vi "POP_Point to Row Col.vi"(8 "error in (no error)":errorcluster, 9 "Point":cluster{"X":i32, "Y":i32}, 11 "Grid Ctl Reference In":refnum<vi>) -> (0 "error out":errorcluster, 1 "Cell Rect Out":T3={"left"=28, "top"=253, "right"=88, "bottom"=213}, 2 "Cell Info Out":T1={"Tag"="", "Row"=0, "Column"=0, "In Symbol?"=FALSE, "In Data?"=FALSE, "Cell String"="", "Ctl Refnum"=refnum, "Prop Type"=enum."Unkown", "Ring Strings"=[], "Ring Values"=[], "New Cell String"=""}, 3 "Grid Ctl Reference Out":refnum<vi>, 4 "In Bounds?":bool)   [LabVIEW 2016]
uses:
  Ctrls/PSPOP_Grid.Cell Info.ctl
  Ctrls/POP_Data Type.ctl
panel:
  in  "Cell Info (type)":T1={"Tag"="", "Row"=0, "Column"=0, "In Symbol?"=FALSE, "In Data?"=FALSE, "Cell String"="", "Ctl Refnum"=refnum, "Prop Type"=enum."Unkown", "Ring Strings"=[], "Ring Values"=[], "New Cell String"=""}
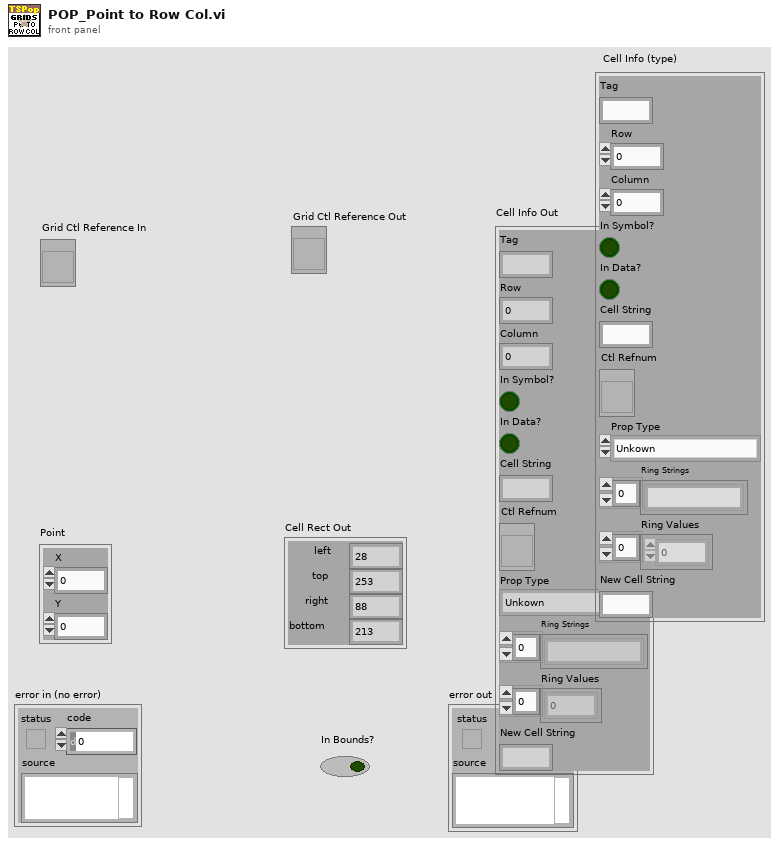
[diagram p1: front panel]
types:
  T1 = typedef "PSPOP_Grid.Cell Info.ctl" = cluster{"Tag":string, "Row":i32, "Column":i32, "In Symbol?":bool, "In Data?":bool, "Cell String":string, "Ctl Refnum":refnum<vi>, "Prop Type":T2, "Ring Strings":string[], "Ring Values":ext[], "New Cell String":string}
  T2 = typedef "POP_Data Type.ctl" = enum16{"NO POPUP", "Unkown", "String", "Integer", "Float", "Color", "Boolean", "Ring", "Captioned String", "Captioned Integer", "Button Color", "2 Int Cluster", "4 Int Cluster", "6-Dbl Cluster", "Path", "Combox", "Time", "ShotCut String"}
  T3 = cluster{"left":i16, "top":i16, "right":i16, "bottom":i16}
  T4 = typedef "LVPositionTypeDef.ctl" = cluster{"Left":i32, "Top":i32}
  T5 = typedef "LVRowAndColumnTypeDef.ctl" = cluster{"Row":i32, "Column":i32}
  T6 = typedef "LVBoundsTypeDef.ctl" = cluster{"Width":u32, "Height":u32}
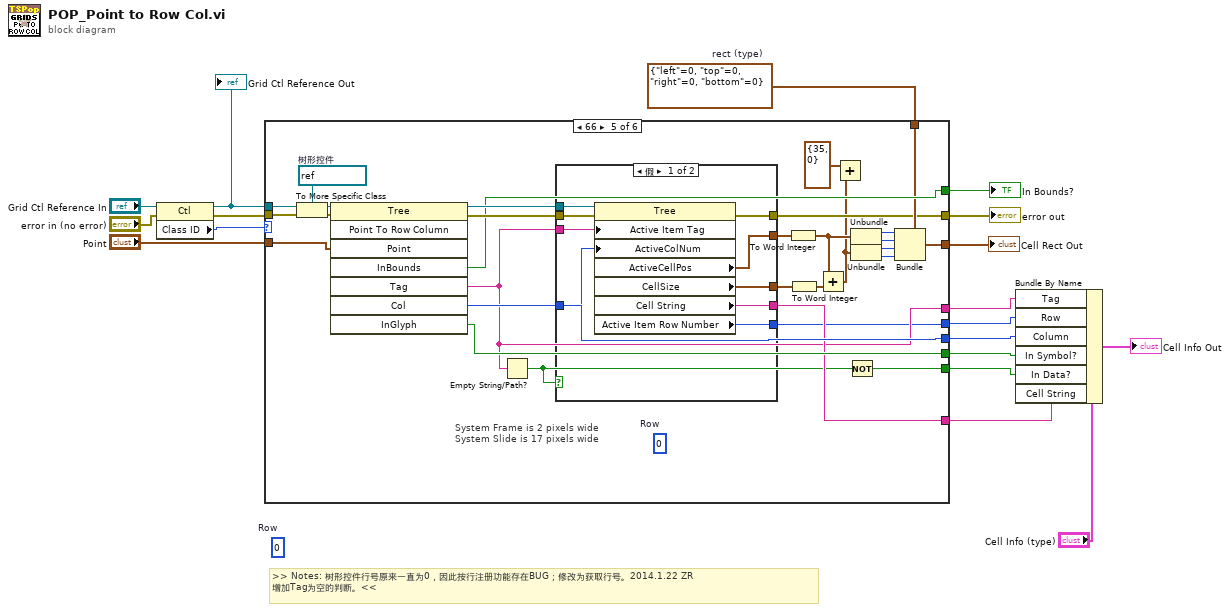
[diagram p0: block diagram]
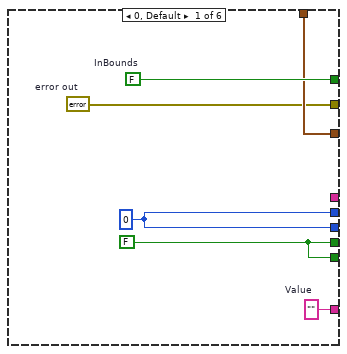
[diagram p2: hidden frame]
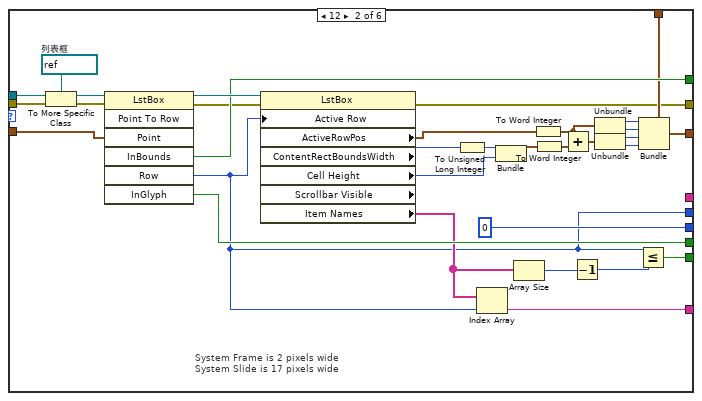
[diagram p3: hidden frame]
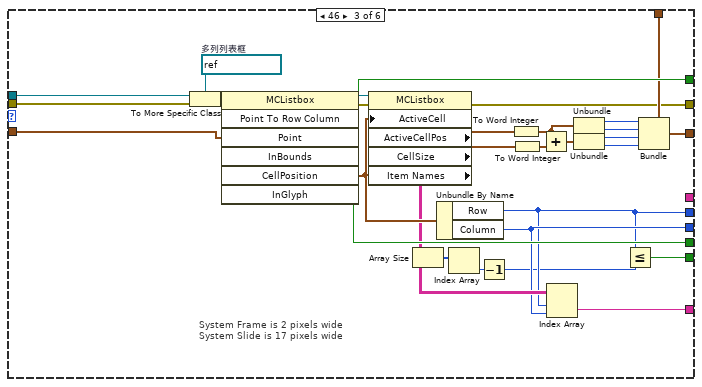
[diagram p4: hidden frame]
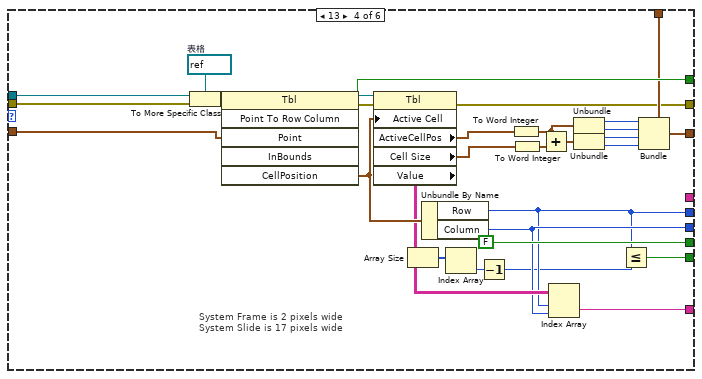
[diagram p5: hidden frame]
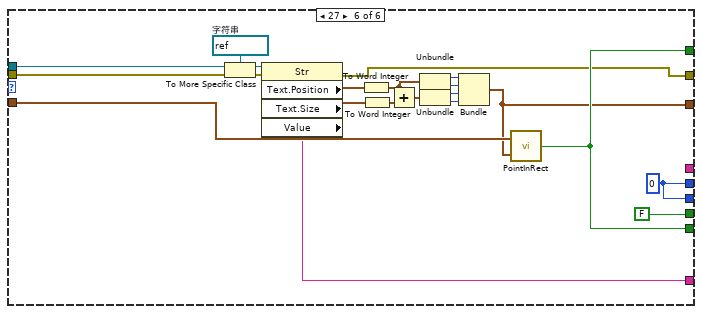
[diagram p7: hidden frame]
diagram:
  (unwired) 0  # Row
  w14 = T3 {"left"=0, "top"=0, "right"=0, "bottom"=0}  # rect (type)
  # ">> Notes: 树形控件行号原来一直为0，因此按行注册功能存在BUG；修改为获取行号。2014.1.22 ZR\n增加Tag为空的判断。<<"
  n1 = property class="Ctl"(reference="Grid Ctl Reference In", error in="error in (no error)") -> (reference out=w2:refnum<vi>, error out=w18:errorcluster, "Class ID"=w8:u32)
  "Grid Ctl Reference Out" <- w2
  n2 = case shown="66" w8 {
    tunnel: w2 -> [_ w55 w86 w117 w146 w164]
    tunnel: w18 -> [_ w54 w85 w116 w145 w163]
    tunnel: [w21 w32 w61 w92 w126 w159] -> w10
    tunnel: "Point" -> [_ w50 w78 w112 w142 w162]
    tunnel: [w23 w31 w60 w91 w120 w178] -> w11
    tunnel: [w23 0 w62 w93 w128 w178] -> w16
    tunnel: [w20 w49 w76 FALSE ("InGlyph") w127 FALSE ("InGlyph")] -> w17
    tunnel: [w22 w35 w66 w95 w129 w158] -> w7
    tunnel: [w24 w48 w77 w109 w139 w161] -> w6
    tunnel: w14 -> [w22 w38 w67 w98 w132 _]
    tunnel: [_ _ _ _ w124 _] -> w12
    tunnel: [w20 w29 w58 w89 w125 w161] -> w9
    tunnel: [w19 w27 w57 w88 w123 w160] -> w3
    frame 0, Default {
      w19 = errorcluster {"status"=TRUE, "code"=1, "source"="Invalid Control"}  # error out
      w21 = ""  # Value
      w20 = FALSE ("InGlyph")
      w24 = FALSE  # InBounds
      w23 = 0
    }
    frame 12 {
      w56 = refnum<vi> refnum  # 列表框
      # "System Frame is 2 pixels wide\nSystem Slide is 17 pixels wide"
      n3 = To More Specific Class(target class=w56, reference=w55, error in=w54) -> (specific class reference=w51:refnum<vi>, error out=w26:errorcluster)
      n4 = invoke class="LstBox" method="Point To Row"(reference=w51, error in=w26, "Point"=w50) -> (reference out=w52:refnum<vi>, error out=w25:errorcluster, "InBounds"=w48:bool, "Row"=w31:i32, "InGlyph"=w49:bool)  [unwired: 4 in, 2 out]
      n5 = property on="Property Node" class="LstBox" props=["Active Row", "ActiveRowPos", "ContentRectBoundsWidth", "Cell Height", "Scrollbar Visible", "Item Names"](reference=w52, error in=w25, "Active Row"=w31) -> (error out=w27:errorcluster, "ActiveRowPos"=w37:T4, "ContentRectBoundsWidth"=w47:i32, "Cell Height"=w46:i32, "Item Names"=w33:string[])  [unwired: 2 out]
      n6 = To Unsigned Long Integer(number=w47) -> (unsigned 32bit integer=w45:u32)
      n7 = Index Array(array=w33, index=w31) -> (element=w32:string)
      n8 = Bundle(w45, "Cell Height"=w46) -> (w36:cluster{u32, "Cell Height":i32})  [unwired: 1 in]
      n9 = Array Size(array=w33) -> (size(s)=w53:i32)
      n10 = To Word Integer(number=w37) -> (16bit integer=w44:cluster{"Left":i16, "Top":i16})
      n11 = To Word Integer(number=w36) -> (16bit integer=w43:cluster{i16, "Cell Height":i16})
      n12 = Add(x=w44, y=w43) -> (x+y=w39:cluster{i16, i16})
      n13 = Decrement(x=w53) -> (x-1=w30:i32)
      n14 = Unbundle(w44) -> ("Left"=w40:i16, "Top"=w41:i16)
      n15 = Unbundle(w39) -> (w28:i16, w42:i16)
      n16 = Less Or Equal?(x=w31, y=w30) -> (x <= y?=w29:bool)
      n17 = Bundle(cluster=w38, "left"=w40, "top"=w41, "right"=w28, "bottom"=w42) -> (w35:T3)
    }
    frame 46 {
      w87 = refnum<vi> refnum  # 多列列表框
      # "System Frame is 2 pixels wide\nSystem Slide is 17 pixels wide"
      n18 = To More Specific Class(target class=w87, reference=w86, error in=w85) -> (specific class reference=w82:refnum<vi>, error out=w81:errorcluster)
      n19 = invoke class="MCListbox" method="Point To Row Column"(reference=w82, error in=w81, "Point"=w78) -> (reference out=w80:refnum<vi>, error out=w79:errorcluster, "InBounds"=w77:bool, "CellPosition"=w75:T5, "InGlyph"=w76:bool)  [unwired: 4 in, 2 out]
      n20 = property on="Property Node" class="MCListbox"(reference=w80, error in=w79, "ActiveCell"=w75) -> (error out=w57:errorcluster, "ActiveCellPos"=w65:T4, "CellSize"=w64:T6, "Item Names"=w63:string[][])  [unwired: 1 out]
      n21 = Array Size(array=w63) -> (size(s)=w84:i32[])
      n22 = Unbundle By Name(w75) -> ("Row"=w60:i32, "Column"=w62:i32)
      n23 = Index Array(array=w84) -> (element=w83:i32)  [unwired: 1 in]
      n24 = Decrement(x=w83) -> (x-1=w59:i32)
      n25 = To Word Integer(number=w65) -> (16bit integer=w74:cluster{"Left":i16, "Top":i16})
      n26 = To Word Integer(number=w64) -> (16bit integer=w73:cluster{"Width":i16, "Height":i16})
      n27 = Add(x=w74, y=w73) -> (x+y=w68:cluster{i16, i16})
      n28 = Index Array(array=w63, index (row)=w60, index (col)=w62) -> (element=w61:string)
      n29 = Unbundle(w74) -> ("Left"=w69:i16, "Top"=w70:i16)
      n30 = Unbundle(w68) -> (w71:i16, w72:i16)
      n31 = Less Or Equal?(x=w60, y=w59) -> (x <= y?=w58:bool)
      n32 = Bundle(cluster=w67, "left"=w69, "top"=w70, "right"=w71, "bottom"=w72) -> (w66:T3)
    }
    frame 13 {
      w118 = refnum<vi> refnum  # 表格
      # "System Frame is 2 pixels wide\nSystem Slide is 17 pixels wide"
      n33 = To More Specific Class(target class=w118, reference=w117, error in=w116) -> (specific class reference=w114:refnum<vi>, error out=w113:errorcluster)
      n34 = invoke class="Tbl" method="Point To Row Column"(reference=w114, error in=w113, "Point"=w112) -> (reference out=w111:refnum<vi>, error out=w110:errorcluster, "InBounds"=w109:bool, "CellPosition"=w106:T5)  [unwired: 3 in, 2 out]
      n35 = property on="Property Node" class="Tbl"(reference=w111, error in=w110, "Active Cell"=w106) -> (error out=w88:errorcluster, "ActiveCellPos"=w97:T4, "Cell Size"=w96:T6, "Value"=w94:string[][])  [unwired: 1 out]
      n36 = Array Size(array=w94) -> (size(s)=w115:i32[])
      n37 = Unbundle By Name(w106) -> ("Row"=w91:i32, "Column"=w93:i32)
      n38 = Index Array(array=w115) -> (element=w108:i32)  [unwired: 1 in]
      n39 = Decrement(x=w108) -> (x-1=w90:i32)
      n40 = To Word Integer(number=w97) -> (16bit integer=w105:cluster{"Left":i16, "Top":i16})
      n41 = To Word Integer(number=w96) -> (16bit integer=w104:cluster{"Width":i16, "Height":i16})
      n42 = Add(x=w105, y=w104) -> (x+y=w99:cluster{i16, i16})
      n43 = Index Array(array=w94, index (row)=w91, index (col)=w93) -> (element=w92:string)
      n44 = Unbundle(w105) -> ("Left"=w100:i16, "Top"=w101:i16)
      n45 = Unbundle(w99) -> (w102:i16, w103:i16)
      n46 = Less Or Equal?(x=w91, y=w90) -> (x <= y?=w89:bool)
      n47 = Bundle(cluster=w98, "left"=w100, "top"=w101, "right"=w102, "bottom"=w103) -> (w95:T3)
    }
    frame 66 {
      (unwired) 0  # Row
      w147 = refnum<vi> refnum  # 树形控件
      # "System Frame is 2 pixels wide\nSystem Slide is 17 pixels wide"
      n48 = To More Specific Class(target class=w147, reference=w146, error in=w145) -> (specific class reference=w144:refnum<vi>, error out=w143:errorcluster)
      n49 = invoke class="Tree" method="Point To Row Column"(reference=w144, error in=w143, "Point"=w142) -> (reference out=w141:refnum<vi>, error out=w140:errorcluster, "InBounds"=w139:bool, "Tag"=w124:string, "Col"=w128:i32, "InGlyph"=w127:bool)  [unwired: 5 in, 2 out]
      n50 = Empty String/Path?(string/path=w124) -> (empty?=w119:bool)
      n51 = case shown="假" w119 {
        tunnel: w141 -> [w156 _]
        tunnel: w140 -> [w155 w157]
        tunnel: [w154 _] -> w131
        tunnel: [w153 _] -> w130
        tunnel: w128 -> [w152 _]
        tunnel: [w151 _] -> w126
        tunnel: w124 -> [w150 _]
        tunnel: [w149 w157] -> w123
        tunnel: [w148 _] -> w120
        frame False {
          n52 = property on="Property Node" class="Tree"(reference=w156, error in=w155, "Active Item Tag"=w150, "ActiveColNum"=w152) -> (error out=w149:errorcluster, "ActiveCellPos"=w154:T4, "CellSize"=w153:T6, "Cell String"=w151:string, "Active Item Row Number"=w148:i32)  [unwired: 1 out]
        }
        frame True {
        }
      }
      n53 = To Word Integer(number=w131) -> (16bit integer=w138:cluster{"Left":i16, "Top":i16})
      n54 = To Word Integer(number=w130) -> (16bit integer=w137:cluster{"Width":i16, "Height":i16})
      n55 = Add(x=w138, y=w137) -> (x+y=w121:cluster{i16, i16})
      n56 = Add(x=cluster{i16, i16} {35, 0}, y=w121) -> ()  [unwired: 1 out]
      n57 = Not(x=w119) -> (.not. x?=w125:bool)
      n58 = Unbundle(w138) -> ("Left"=w133:i16, "Top"=w134:i16)
      n59 = Unbundle(w121) -> (w135:i16, w136:i16)
      n60 = Bundle(cluster=w132, "left"=w133, "top"=w134, "right"=w135, "bottom"=w136) -> (w129:T3)
    }
    frame 27 {
      w165 = refnum<vi> refnum  # 字符串
      w178 = 0 ("Row")
      n61 = To More Specific Class(target class=w165, reference=w164, error in=w163) -> (specific class reference=w166:refnum<vi>, error out=w167:errorcluster)
      n62 = property class="Str"(reference=w166, error in=w167) -> (error out=w160:errorcluster, "Text.Position"=w168:T4, "Text.Size"=w169:T6, "Value"=w159:string)  [unwired: 1 out]
      n63 = To Word Integer(number=w168) -> (16bit integer=w176:cluster{"Left":i16, "Top":i16})
      n64 = To Word Integer(number=w169) -> (16bit integer=w170:cluster{"Width":i16, "Height":i16})
      n65 = Add(x=w176, y=w170) -> (x+y=w175:cluster{i16, i16})
      n66 = Unbundle(w176) -> ("Left"=w174:i16, "Top"=w173:i16)
      n67 = Unbundle(w175) -> (w172:i16, w171:i16)
      n68 = Bundle("Left"=w174, "Top"=w173, w172, w171) -> (w158:cluster{"Left":i16, "Top":i16, i16, i16})  [unwired: 1 in]
      n69 = call <vilib>:"PointInRect.vi"("rect"=w158, "point"=w162) -> ("pt in rect"=w161:bool)
    }
  }
  "In Bounds?" <- w6
  "error out" <- w3
  "Cell Rect Out" <- w7
  n70 = Bundle By Name(cluster="Cell Info (type)", "Tag"=w12, "Row"=w11, "Column"=w16, "In Symbol?"=w17, "In Data?"=w9, "Cell String"=w10) -> (→"Cell Info Out":T1)
